vi "Get Active List - By Channel Number.vi"(7 "Parameters Array (in)":T1[](array[typedef])) -> (8 "Active Channel Numbers":i32[](array[numeric]))   [LabVIEW 2017] (continued)
"Default Value"="0"}, {"Core Number"=0, "Channel Number"=19, "Channel Name"="ENG_LB2", "Channel Speed"=100, "Label Decimal"=121, "Label Name"="Label_171", "Min Rate (mS)"=800, "Max Rate (mS)"=1200, "SDI"=0, "SSM"=3, "Create SDI"=FALSE, "Create SSM"=FALSE, "Create Parity"=FALSE, "Parameter Name"="eng_lb2_lbl171_b14_27", "Start Bit"=14, "Number of Bits"=14, "Scale"="0.015625", "Offset"="0", "Signed"=FALSE, "Unit"="% Shaftspeed", "Encoding"=enum."BNR", "Default Value"="0"}, {"Core Number"=0, "Channel Number"=19, "Channel Name"="ENG_LB2", "Channel Speed"=100, "Label Decimal"=122, "Label Name"="Label_172", "Min Rate (mS)"=800, "Max Rate (mS)"=1200, "SDI"=0, "SSM"=3, "Create SDI"=FALSE, "Create SSM"=FALSE, "Create Parity"=FALSE, "Parameter Name"="eng_lb2_lbl172_b14_27", "Start Bit"=14, "Number of Bits"=14, "Scale"="0.015625", "Offset"="0", "Signed"=FALSE, "Unit"="% Shaftspeed", "Encoding"=enum."BNR", "Default Value"="0"}, {"Core Number"=0, "Channel Number"=19, "Channel Name"="ENG_LB2", "Channel Speed"=100, "Label Decimal"=123, "Label Name"="Label_173", "Min Rate (mS)"=800, "Max Rate (mS)"=1200, "SDI"=0, "SSM"=3, "Create SDI"=FALSE, "Create SSM"=FALSE, "Create Parity"=FALSE, "Parameter Name"="eng_lb2_lbl173_b14_27", "Start Bit"=14, "Number of Bits"=14, "Scale"="0.015625", "Offset"="0", "Signed"=FALSE, "Unit"="% Shaftspeed", "Encoding"=enum."BNR", "Default Value"="0"}, {"Core Number"=0, "Channel Number"=19, "Channel Name"="ENG_LB2", "Channel Speed"=100, "Label Decimal"=124, "Label Name"="Label_174", "Min Rate (mS)"=800, "Max Rate (mS)"=1200, "SDI"=0, "SSM"=3, "Create SDI"=FALSE, "Create SSM"=FALSE, "Create Parity"=FALSE, "Parameter Name"="eng_lb2_lbl174_b14_27", "Start Bit"=14, "Number of Bits"=14, "Scale"="0.015625", "Offset"="0", "Signed"=FALSE, "Unit"="% Shaftspeed", "Encoding"=enum."BNR", "Default Value"="0"}, {"Core Number"=0, "Channel Number"=19, "Channel Name"="ENG_LB2", "Channel Speed"=100, "Label Decimal"=128, "Label Name"="Label_200", "Min Rate (mS)"=800, "Max Rate (mS)"=1200, "SDI"=0, "SSM"=3, "Create SDI"=FALSE, "Create SSM"=FALSE, "Create Parity"=FALSE, "Parameter Name"="eng_lb2_lbl200_b16_28", "Start Bit"=16, "Number of Bits"=13, "Scale"="0.125", "Offset"="0", "Signed"=TRUE, "Unit"="Degrees C", "Encoding"=enum."BNR", "Default Value"="0"}, {"Core Number"=0, "Channel Number"=19, "Channel Name"="ENG_LB2", "Channel Speed"=100, "Label Decimal"=160, "Label Name"="Label_240", "Min Rate (mS)"=800, "Max Rate (mS)"=1200, "SDI"=0, "SSM"=3, "Create SDI"=FALSE, "Create SSM"=FALSE, "Create Parity"=FALSE, "Parameter Name"="eng_lb2_lbl240_b15_28", "Start Bit"=15, "Number of Bits"=14, "Scale"="0.5", "Offset"="0", "Signed"=TRUE, "Unit"="Degrees C", "Encoding"=enum."BNR", "Default Value"="0"}, {"Core Number"=0, "Channel Number"=19, "Channel Name"="ENG_LB2", "Channel Speed"=100, "Label Decimal"=163, "Label Name"="Label_243", "Min Rate (mS)"=800, "Max Rate (mS)"=1200, "SDI"=0, "SSM"=3, "Create SDI"=FALSE, "Create SSM"=FALSE, "Create Parity"=FALSE, "Parameter Name"="eng_lb2_lbl243_b15_28", "Start Bit"=15, "Number of Bits"=14, "Scale"="0.5", "Offset"="0", "Signed"=TRUE, "Unit"="Degrees C", "Encoding"=enum."BNR", "Default Value"="0"}, {"Core Number"=0, "Channel Number"=19, "Channel Name"="ENG_LB2", "Channel Speed"=100, "Label Decimal"=72, "Label Name"="Label_110", "Min Rate (mS)"=800, "Max Rate (mS)"=1200, "SDI"=0, "SSM"=3, "Create SDI"=FALSE, "Create SSM"=FALSE, "Create Parity"=FALSE, "Parameter Name"="eng_lb2_lbl110_b20_28", "Start Bit"=20, "Number of Bits"=9, "Scale"="2", "Offset"="0", "Signed"=TRUE, "Unit"="Psig", "Encoding"=enum."BNR", "Default Value"="0"}, {"Core Number"=0, "Channel Number"=19, "Channel Name"="ENG_LB2", "Channel Speed"=100, "Label Decimal"=89, "Label Name"="Label_131", "Min Rate (mS)"=800, "Max Rate (mS)"=1200, "SDI"=0, "SSM"=3, "Create SDI"=FALSE, "Create SSM"=FALSE, "Create Parity"=FALSE, "Parameter Name"="eng_lb2_lbl131_b15_27", "Start Bit"=15, "Number of Bits"=13, "Scale"="0.015625", "Offset"="0", "Signed"=FALSE, "Unit"="Psid", "Encoding"=enum."BNR", "Default Value"="0"}, {"Core Number"=0, "Channel Number"=19, "Channel Name"="ENG_LB2", "Channel Speed"=100, "Label Decimal"=137, "Label Name"="Label_211", "Min Rate (mS)"=800, "Max Rate (mS)"=1200, "SDI"=0, "SSM"=3, "Create SDI"=FALSE, "Create SSM"=FALSE, "Create Parity"=FALSE, "Parameter Name"="eng_lb2_lbl211_b20_28", "Start Bit"=20, "Number of Bits"=9, "Scale"="0.25", "Offset"="0", "Signed"=TRUE, "Unit"="Psid", "Encoding"=enum."BNR", "Default Value"="0"}, {"Core Number"=0, "Channel Number"=19, "Channel Name"="ENG_LB2", "Channel Speed"=100, "Label Decimal"=92, "Label Name"="Label_134", "Min Rate (mS)"=800, "Max Rate (mS)"=1200, "SDI"=0, "SSM"=3, "Create SDI"=FALSE, "Create SSM"=FALSE, "Create Parity"=FALSE, "Parameter Name"="eng_lb2_lbl134_b13_28", "Start Bit"=13, "Number of Bits"=16, "Scale"="0.03125", "Offset"="0", "Signed"=TRUE, "Unit"="Degrees", "Encoding"=enum."BNR", "Default Value"="0"}, {"Core Number"=0, "Channel Number"=19, "Channel Name"="ENG_LB2", "Channel Speed"=100, "Label Decimal"=60, "Label Name"="Label_74", "Min Rate (mS)"=800, "Max Rate (mS)"=1200, "SDI"=0, "SSM"=3, "Create SDI"=FALSE, "Create SSM"=FALSE, "Create Parity"=FALSE, "Parameter Name"="eng_lb2_lbl74_b15_28", "Start Bit"=15, "Number of Bits"=14, "Scale"="0.00390625", "Offset"="0", "Signed"=TRUE, "Unit"="US pints below full", "Encoding"=enum."BNR", "Default Value"="0"}, {"Core Number"=0, "Channel Number"=19, "Channel Name"="ENG_LB2", "Channel Speed"=100, "Label Decimal"=196, "Label Name"="Label_304", "Min Rate (mS)"=800, "Max Rate (mS)"=1200, "SDI"=0, "SSM"=3, "Create SDI"=FALSE, "Create SSM"=FALSE, "Create Parity"=FALSE, "Parameter Name"="eng_lb2_lbl304_b14_28", "Start Bit"=14, "Number of Bits"=15, "Scale"="0.0078125", "Offset"="0", "Signed"=TRUE, "Unit"="Psid", "Encoding"=enum."BNR", "Default Value"="0"}, {"Core Number"=0, "Channel Number"=19, "Channel Name"="ENG_LB2", "Channel Speed"=100, "Label Decimal"=170, "Label Name"="Label_252", "Min Rate (mS)"=800, "Max Rate (mS)"=1200, "SDI"=0, "SSM"=3, "Create SDI"=FALSE, "Create SSM"=FALSE, "Create Parity"=FALSE, "Parameter Name"="eng_lb2_lbl252_b16_27", "Start Bit"=16, "Number of Bits"=12, "Scale"="0.0009765625", "Offset"="0", "Signed"=FALSE, "Unit"="Pressure ratio", "Encoding"=enum."BNR", "Default Value"="0"}, {"Core Number"=0, "Channel Number"=19, "Channel Name"="ENG_LB2", "Channel Speed"=100, "Label Decimal"=48, "Label Name"="Label_60", "Min Rate (mS)"=800, "Max Rate (mS)"=1200, "SDI"=0, "SSM"=3, "Create SDI"=FALSE, "Create SSM"=FALSE, "Create Parity"=FALSE, "Parameter Name"="eng_lb2_lbl60_b13_27", "Start Bit"=13, "Number of Bits"=15, "Scale"="1", "Offset"="0", "Signed"=FALSE, "Unit"="N/A", "Encoding"=enum."BNR", "Default Value"="0"}, {"Core Number"=0, "Channel Number"=19, "Channel Name"="ENG_LB2", "Channel Speed"=100, "Label Decimal"=150, "Label Name"="Label_226", "Min Rate (mS)"=800, "Max Rate (mS)"=1200, "SDI"=0, "SSM"=3, "Create SDI"=FALSE, "Create SSM"=FALSE, "Create Parity"=FALSE, "Parameter Name"="eng_lb2_lbl226_b13_27", "Start Bit"=13, "Number of Bits"=15, "Scale"="1", "Offset"="0", "Signed"=FALSE, "Unit"="N/A", "Encoding"=enum."BNR", "Default Value"="0"}, {"Core Number"=0, "Channel Number"=19, "Channel Name"="ENG_LB2", "Channel Speed"=100, "Label Decimal"=151, "Label Name"="Label_227", "Min Rate (mS)"=800, "Max Rate (mS)"=1200, "SDI"=0, "SSM"=3, "Create SDI"=FALSE, "Create SSM"=FALSE, "Create Parity"=FALSE, "Parameter Name"="eng_lb2_lbl227_b13_27", "Start Bit"=13, "Number of Bits"=15, "Scale"="1", "Offset"="0", "Signed"=FALSE, "Unit"="N/A", "Encoding"=enum."BNR", "Default Value"="0"}, {"Core Number"=0, "Channel Number"=19, "Channel Name"="ENG_LB2", "Channel Speed"=100, "Label Decimal"=158, "Label Name"="Label_236", "Min Rate (mS)"=800, "Max Rate (mS)"=1200, "SDI"=0, "SSM"=3, "Create SDI"=FALSE, "Create SSM"=FALSE, "Create Parity"=FALSE, "Parameter Name"="eng_lb2_lbl236_b13_27", "Start Bit"=13, "Number of Bits"=15, "Scale"="1", "Offset"="0", "Signed"=FALSE, "Unit"="N/A", "Encoding"=enum."BNR", "Default Value"="0"}, {"Core Number"=0, "Channel Number"=19, "Channel Name"="ENG_LB2", "Channel Speed"=100, "Label Decimal"=184, "Label Name"="Label_270", "Min Rate (mS)"=40, "Max Rate (mS)"=60, "SDI"=0, "SSM"=0, "Create SDI"=FALSE, "Create SSM"=FALSE, "Create Parity"=FALSE, "Parameter Name"="eng_lb2_lbl270_b10_28", "Start Bit"=10, "Number of Bits"=19, "Scale"="1", "Offset"="0", "Signed"=FALSE, "Unit"="N/A", "Encoding"=enum."Discrete", "Default Value"="0"}, {"Core Number"=0, "Channel Number"=19, "Channel Name"="ENG_LB2", "Channel Speed"=100, "Label Decimal"=232, "Label Name"="Label_350", "Min Rate (mS)"=160, "Max Rate (mS)"=240, "SDI"=0, "SSM"=0, "Create SDI"=FALSE, "Create SSM"=FALSE, "Create Parity"=FALSE, "Parameter Name"="eng_lb2_lbl350_b10_28", "Start Bit"=10, "Number of Bits"=19, "Scale"="1", "Offset"="0", "Signed"=FALSE, "Unit"="N/A", "Encoding"=enum."Discrete", "Default Value"="0"}, {"Core Number"=0, "Channel Number"=19, "Channel Name"="ENG_LB2", "Channel Speed"=100, "Label Decimal"=185, "Label Name"="Label_271", "Min Rate (mS)"=160, "Max Rate (mS)"=240, "SDI"=0, "SSM"=0, "Create SDI"=FALSE, "Create SSM"=FALSE, "Create Parity"=FALSE, "Parameter Name"="eng_lb2_lbl271_b10_28", "Start Bit"=10, "Number of Bits"=19, "Scale"="1", "Offset"="0", "Signed"=FALSE, "Unit"="N/A", "Encoding"=enum."Discrete", "Default Value"="0"}, {"Core Number"=0, "Channel Number"=19, "Channel Name"="ENG_LB2", "Channel Speed"=100, "Label Decimal"=186, "Label Name"="Label_272", "Min Rate (mS)"=160, "Max Rate (mS)"=240, "SDI"=0, "SSM"=0, "Create SDI"=FALSE, "Create SSM"=FALSE, "Create Parity"=FALSE, "Parameter Name"="eng_lb2_lbl272_b10_28", "Start Bit"=10, "Number of Bits"=19, "Scale"="1", "Offset"="0", "Signed"=FALSE, "Unit"="N/A", "Encoding"=enum."Discrete", "Default Value"="0"}, {"Core Number"=0, "Channel Number"=19, "Channel Name"="ENG_LB2", "Channel Speed"=100, "Label Decimal"=187, "Label Name"="Label_273", "Min Rate (mS)"=160, "Max Rate (mS)"=240, "SDI"=0, "SSM"=0, "Create SDI"=FALSE, "Create SSM"=FALSE, "Create Parity"=FALSE, "Parameter Name"="eng_lb2_lbl273_b10_28", "Start Bit"=10, "Number of Bits"=19, "Scale"="1", "Offset"="0", "Signed"=FALSE, "Unit"="N/A", "Encoding"=enum."Discrete", "Default Value"="0"}, {"Core Number"=0, "Channel Number"=19, "Channel Name"="ENG_LB2", "Channel Speed"=100, "Label Decimal"=188, "Label Name"="Label_274", "Min Rate (mS)"=160, "Max Rate (mS)"=240, "SDI"=0, "SSM"=0, "Create SDI"=FALSE, "Create SSM"=FALSE, "Create Parity"=FALSE, "Parameter Name"="eng_lb2_lbl274_b10_28", "Start Bit"=10, "Number of Bits"=19, "Scale"="1", "Offset"="0", "Signed"=FALSE, "Unit"="N/A", "Encoding"=enum."Discrete", "Default Value"="0"}, {"Core Number"=0, "Channel Number"=19, "Channel Name"="ENG_LB2", "Channel Speed"=100, "Label Decimal"=189, "Label Name"="Label_275", "Min Rate (mS)"=160, "Max Rate (mS)"=240, "SDI"=0, "SSM"=0, "Create SDI"=FALSE, "Create SSM"=FALSE, "Create Parity"=FALSE, "Parameter Name"="eng_lb2_lbl275_b10_28", "Start Bit"=10, "Number of Bits"=19, "Scale"="1", "Offset"="0", "Signed"=FALSE, "Unit"="N/A", "Encoding"=enum."Discrete", "Default Value"="0"}, {"Core Number"=0, "Channel Number"=19, "Channel Name"="ENG_LB2", "Channel Speed"=100, "Label Decimal"=190, "Label Name"="Label_276", "Min Rate (mS)"=160, "Max Rate (mS)"=240, "SDI"=0, "SSM"=0, "Create SDI"=FALSE, "Create SSM"=FALSE, "Create Parity"=FALSE, "Parameter Name"="eng_lb2_lbl276_b10_28", "Start Bit"=10, "Number of Bits"=19, "Scale"="1", "Offset"="0", "Signed"=FALSE, "Unit"="N/A", "Encoding"=enum."Discrete", "Default Value"="0"}, {"Core Number"=0, "Channel Number"=19, "Channel Name"="ENG_LB2", "Channel Speed"=100, "Label Decimal"=191, "Label Name"="Label_277", "Min Rate (mS)"=160, "Max Rate (mS)"=240, "SDI"=0, "SSM"=0, "Create SDI"=FALSE, "Create SSM"=FALSE, "Create Parity"=FALSE, "Parameter Name"="eng_lb2_lbl277_b10_28", "Start Bit"=10, "Number of Bits"=19, "Scale"="1", "Offset"="0", "Signed"=FALSE, "Unit"="N/A", "Encoding"=enum."Discrete", "Default Value"="0"}, {"Core Number"=0, "Channel Number"=19, "Channel Name"="ENG_LB2", "Channel Speed"=100, "Label Decimal"=254, "Label Name"="Label_376", "Min Rate (mS)"=160, "Max Rate (mS)"=240, "SDI"=0, "SSM"=0, "Create SDI"=FALSE, "Create SSM"=FALSE, "Create Parity"=FALSE, "Parameter Name"="eng_lb2_lbl376_b10_28", "Start Bit"=10, "Number of Bits"=19, "Scale"="1", "Offset"="0", "Signed"=FALSE, "Unit"="N/A", "Encoding"=enum."Discrete", "Default Value"="0"}, {"Core Number"=0, "Channel Number"=19, "Channel Name"="ENG_LB2", "Channel Speed"=100, "Label Decimal"=104, "Label Name"="Label_150", "Min Rate (mS)"=720, "Max Rate (mS)"=1080, "SDI"=0, "SSM"=0, "Create SDI"=FALSE, "Create SSM"=FALSE, "Create Parity"=FALSE, "Parameter Name"="eng_lb2_lbl150_b10_28", "Start Bit"=10, "Number of Bits"=19, "Scale"="1", "Offset"="0", "Signed"=FALSE, "Unit"="N/A", "Encoding"=enum."Discrete", "Default Value"="0"}, {"Core Number"=0, "Channel Number"=19, "Channel Name"="ENG_LB2", "Channel Speed"=100, "Label Decimal"=105, "Label Name"="Label_151", "Min Rate (mS)"=720, "Max Rate (mS)"=1080, "SDI"=0, "SSM"=0, "Create SDI"=FALSE, "Create SSM"=FALSE, "Create Parity"=FALSE, "Parameter Name"="eng_lb2_lbl151_b10_28", "Start Bit"=10, "Number of Bits"=19, "Scale"="1", "Offset"="0", "Signed"=FALSE, "Unit"="N/A", "Encoding"=enum."Discrete", "Default Value"="0"}, {"Core Number"=0, "Channel Number"=19, "Channel Name"="ENG_LB2", "Channel Speed"=100, "Label Decimal"=107, "Label Name"="Label_153", "Min Rate (mS)"=720, "Max Rate (mS)"=1080, "SDI"=0, "SSM"=0, "Create SDI"=FALSE, "Create SSM"=FALSE, "Create Parity"=FALSE, "Parameter Name"="eng_lb2_lbl153_b10_28", "Start Bit"=10, "Number of Bits"=19, "Scale"="1", "Offset"="0", "Signed"=FALSE, "Unit"="N/A", "Encoding"=enum."Discrete", "Default Value"="0"}, {"Core Number"=0, "Channel Number"=19, "Channel Name"="ENG_LB2", "Channel Speed"=100, "Label Decimal"=108, "Label Name"="Label_154", "Min Rate (mS)"=720, "Max Rate (mS)"=1080, "SDI"=0, "SSM"=0, "Create SDI"=FALSE, "Create SSM"=FALSE, "Create Parity"=FALSE, "Parameter Name"="eng_lb2_lbl154_b10_28", "Start Bit"=10, "Number of Bits"=19, "Scale"="1", "Offset"="0", "Signed"=FALSE, "Unit"="N/A", "Encoding"=enum."Discrete", "Default Value"="0"}, {"Core Number"=0, "Channel Number"=19, "Channel Name"="ENG_LB2", "Channel Speed"=100, "Label Decimal"=109, "Label Name"="Label_155", "Min Rate (mS)"=720, "Max Rate (mS)"=1080, "SDI"=0, "SSM"=0, "Create SDI"=FALSE, "Create SSM"=FALSE, "Create Parity"=FALSE, "Parameter Name"="eng_lb2_lbl155_b10_28", "Start Bit"=10, "Number of Bits"=19, "Scale"="1", "Offset"="0", "Signed"=FALSE, "Unit"="N/A", "Encoding"=enum."Discrete", "Default Value"="0"}, {"Core Number"=0, "Channel Number"=19, "Channel Name"="ENG_LB2", "Channel Speed"=100, "Label Decimal"=110, "Label Name"="Label_156", "Min Rate (mS)"=720, "Max Rate (mS)"=1080, "SDI"=0, "SSM"=0, "Create SDI"=FALSE, "Create SSM"=FALSE, "Create Parity"=FALSE, "Parameter Name"="eng_lb2_lbl156_b10_28", "Start Bit"=10, "Number of Bits"=19, "Scale"="1", "Offset"="0", "Signed"=FALSE, "Unit"="N/A", "Encoding"=enum."Discrete", "Default Value"="0"}, {"Core Number"=0, "Channel Number"=19, "Channel Name"="ENG_LB2", "Channel Speed"=100, "Label Decimal"=111, "Label Name"="Label_157", "Min Rate (mS)"=720, "Max Rate (mS)"=1080, "SDI"=0, "SSM"=0, "Create SDI"=FALSE, "Create SSM"=FALSE, "Create Parity"=FALSE, "Parameter Name"="eng_lb2_lbl157_b10_28", "Start Bit"=10, "Number of Bits"=19, "Scale"="1", "Offset"="0", "Signed"=FALSE, "Unit"="N/A", "Encoding"=enum."Discrete", "Default Value"="0"}, {"Core Number"=0, "Channel Number"=19, "Channel Name"="ENG_LB2", "Channel Speed"=100, "Label Decimal"=112, "Label Name"="Label_160", "Min Rate (mS)"=720, "Max Rate (mS)"=1080, "SDI"=0, "SSM"=0, "Create SDI"=FALSE, "Create SSM"=FALSE, "Create Parity"=FALSE, "Parameter Name"="eng_lb2_lbl160_b10_28", "Start Bit"=10, "Number of Bits"=19, "Scale"="1", "Offset"="0", "Signed"=FALSE, "Unit"="N/A", "Encoding"=enum."Discrete", "Default Value"="0"}, {"Core Number"=0, "Channel Number"=19, "Channel Name"="ENG_LB2", "Channel Speed"=100, "Label Decimal"=113, "Label Name"="Label_161", "Min Rate (mS)"=720, "Max Rate (mS)"=1080, "SDI"=0, "SSM"=0, "Create SDI"=FALSE, "Create SSM"=FALSE, "Create Parity"=FALSE, "Parameter Name"="eng_lb2_lbl161_b10_28", "Start Bit"=10, "Number of Bits"=19, "Scale"="1", "Offset"="0", "Signed"=FALSE, "Unit"="N/A", "Encoding"=enum."Discrete", "Default Value"="0"}, {"Core Number"=0, "Channel Number"=19, "Channel Name"="ENG_LB2", "Channel Speed"=100, "Label Decimal"=114, "Label Name"="Label_162", "Min Rate (mS)"=720, "Max Rate (mS)"=1080, "SDI"=0, "SSM"=0, "Create SDI"=FALSE, "Create SSM"=FALSE, "Create Parity"=FALSE, "Parameter Name"="eng_lb2_lbl162_b10_28", "Start Bit"=10, "Number of Bits"=19, "Scale"="1", "Offset"="0", "Signed"=FALSE, "Unit"="N/A", "Encoding"=enum."Discrete", "Default Value"="0"}, {"Core Number"=0, "Channel Number"=19, "Channel Name"="ENG_LB2", "Channel Speed"=100, "Label Decimal"=115, "Label Name"="Label_163", "Min Rate (mS)"=720, "Max Rate (mS)"=1080, "SDI"=0, "SSM"=0, "Create SDI"=FALSE, "Create SSM"=FALSE, "Create Parity"=FALSE, "Parameter Name"="eng_lb2_lbl163_b10_28", "Start Bit"=10, "Number of Bits"=19, "Scale"="1", "Offset"="0", "Signed"=FALSE, "Unit"="N/A", "Encoding"=enum."Discrete", "Default Value"="0"}, {"Core Number"=0, "Channel Number"=19, "Channel Name"="ENG_LB2", "Channel Speed"=100, "Label Decimal"=117, "Label Name"="Label_165", "Min Rate (mS)"=720, "Max Rate (mS)"=1080, "SDI"=0, "SSM"=0, "Create SDI"=FALSE, "Create SSM"=FALSE, "Create Parity"=FALSE, "Parameter Name"="eng_lb2_lbl165_b10_28", "Start Bit"=10, "Number of Bits"=19, "Scale"="1", "Offset"="0", "Signed"=FALSE, "Unit"="N/A", "Encoding"=enum."Discrete", "Default Value"="0"}, {"Core Number"=0, "Channel Number"=19, "Channel Name"="ENG_LB2", "Channel Speed"=100, "Label Decimal"=119, "Label Name"="Label_167", "Min Rate (mS)"=720, "Max Rate (mS)"=1080, "SDI"=0, "SSM"=0, "Create SDI"=FALSE, "Create SSM"=FALSE, "Create Parity"=FALSE, "Parameter Name"="eng_lb2_lbl167_b10_28", "Start Bit"=10, "Number of Bits"=19, "Scale"="1", "Offset"="0", "Signed"=FALSE, "Unit"="N/A", "Encoding"=enum."Discrete", "Default Value"="0"}, {"Core Number"=0, "Channel Number"=19, "Channel Name"="ENG_LB2", "Channel Speed"=100, "Label Decimal"=120, "Label Name"="Label_170", "Min Rate (mS)"=720, "Max Rate (mS)"=1080, "SDI"=0, "SSM"=0, "Create SDI"=FALSE, "Create SSM"=FALSE, "Create Parity"=FALSE, "Parameter Name"="eng_lb2_lbl170_b10_28", "Start Bit"=10, "Number of Bits"=19, "Scale"="1", "Offset"="0", "Signed"=FALSE, "Unit"="N/A", "Encoding"=enum."Discrete", "Default Value"="0"}, {"Core Number"=0, "Channel Number"=19, "Channel Name"="ENG_LB2", "Channel Speed"=100, "Label Decimal"=125, "Label Name"="Label_175", "Min Rate (mS)"=720, "Max Rate (mS)"=1080, "SDI"=0, "SSM"=0, "Create SDI"=FALSE, "Create SSM"=FALSE, "Create Parity"=FALSE, "Parameter Name"="eng_lb2_lbl175_b10_28", "Start Bit"=10, "Number of Bits"=19, "Scale"="1", "Offset"="0", "Signed"=FALSE, "Unit"="N/A", "Encoding"=enum."Discrete", "Default Value"="0"}, {"Core Number"=0, "Channel Number"=19, "Channel Name"="ENG_LB2", "Channel Speed"=100, "Label Decimal"=126, "Label Name"="Label_176", "Min Rate (mS)"=720, "Max Rate (mS)"=1080, "SDI"=0, "SSM"=0, "Create SDI"=FALSE, "Create SSM"=FALSE, "Create Parity"=FALSE, "Parameter Name"="eng_lb2_lbl176_b10_28", "Start Bit"=10, "Number of Bits"=19, "Scale"="1", "Offset"="0", "Signed"=FALSE, "Unit"="N/A", "Encoding"=enum."Discrete", "Default Value"="0"}, {"Core Number"=0, "Channel Number"=19, "Channel Name"="ENG_LB2", "Channel Speed"=100, "Label Decimal"=127, "Label Name"="Label_177", "Min Rate (mS)"=720, "Max Rate (mS)"=1080, "SDI"=0, "SSM"=0, "Create SDI"=FALSE, "Create SSM"=FALSE, "Create Parity"=FALSE, "Parameter Name"="eng_lb2_lbl177_b10_28", "Start Bit"=10, "Number of Bits"=19, "Scale"="1", "Offset"="0", "Signed"=FALSE, "Unit"="N/A", "Encoding"=enum."Discrete", "Default Value"="0"}, {"Core Number"=0, "Channel Number"=19, "Channel Name"="ENG_LB2", "Channel Speed"=100, "Label Decimal"=129, "Label Name"="Label_201", "Min Rate (mS)"=720, "Max Rate (mS)"=1080, "SDI"=0, "SSM"=0, "Create SDI"=FALSE, "Create SSM"=FALSE, "Create Parity"=FALSE, "Parameter Name"="eng_lb2_lbl201_b10_28", "Start Bit"=10, "Number of Bits"=19, "Scale"="1", "Offset"="0", "Signed"=FALSE, "Unit"="N/A", "Encoding"=enum."Discrete", "Default Value"="0"}, {"Core Number"=0, "Channel Number"=19, "Channel Name"="ENG_LB2", "Channel Speed"=100, "Label Decimal"=130, "Label Name"="Label_202", "Min Rate (mS)"=720, "Max Rate (mS)"=1080, "SDI"=0, "SSM"=0, "Create SDI"=FALSE, "Create SSM"=FALSE, "Create Parity"=FALSE, "Parameter Name"="eng_lb2_lbl202_b10_28", "Start Bit"=10, "Number of Bits"=19, "Scale"="1", "Offset"="0", "Signed"=FALSE, "Unit"="N/A", "Encoding"=enum."Discrete", "Default Value"="0"}, {"Core Number"=0, "Channel Number"=19, "Channel Name"="ENG_LB2", "Channel Speed"=100, "Label Decimal"=132, "Label Name"="Label_204", "Min Rate (mS)"=720, "Max Rate (mS)"=1080, "SDI"=0, "SSM"=0, "Create SDI"=FALSE, "Create SSM"=FALSE, "Create Parity"=FALSE, "Parameter Name"="eng_lb2_lbl204_b10_28", "Start Bit"=10, "Number of Bits"=19, "Scale"="1", "Offset"="0", "Signed"=FALSE, "Unit"="N/A", "Encoding"=enum."Discrete", "Default Value"="0"}, {"Core Number"=0, "Channel Number"=19, "Channel Name"="ENG_LB2", "Channel Speed"=100, "Label Decimal"=139, "Label Name"="Label_213", "Min Rate (mS)"=800, "Max Rate (mS)"=1200, "SDI"=0, "SSM"=0, "Create SDI"=FALSE, "Create SSM"=FALSE, "Create Parity"=FALSE, "Parameter Name"="eng_lb2_lbl213_b10_28", "Start Bit"=10, "Number of Bits"=19, "Scale"="1", "Offset"="0", "Signed"=FALSE, "Unit"="N/A", "Encoding"=enum."Discrete", "Default Value"="0"}, {"Core Number"=0, "Channel Number"=19, "Channel Name"="ENG_LB2", "Channel Speed"=100, "Label Decimal"=64, "Label Name"="Label_100", "Min Rate (mS)"=800, "Max Rate (mS)"=1200, "SDI"=0, "SSM"=0, "Create SDI"=FALSE, "Create SSM"=FALSE, "Create Parity"=FALSE, "Parameter Name"="eng_lb2_lbl100_b13_27", "Start Bit"=13, "Number of Bits"=15, "Scale"="1", "Offset"="0", "Signed"=FALSE, "Unit"="N/A", "Encoding"=enum."Discrete", "Default Value"="0"}, {"Core Number"=0, "Channel Number"=19, "Channel Name"="ENG_LB2", "Channel Speed"=100, "Label Decimal"=66, "Label Name"="Label_102", "Min Rate (mS)"=800, "Max Rate (mS)"=1200, "SDI"=0, "SSM"=0, "Create SDI"=FALSE, "Create SSM"=FALSE, "Create Parity"=FALSE, "Parameter Name"="eng_lb2_lbl102_b13_27", "Start Bit"=13, "Number of Bits"=15, "Scale"="1", "Offset"="0", "Signed"=FALSE, "Unit"="N/A", "Encoding"=enum."Discrete", "Default Value"="0"}, {"Core Number"=0, "Channel Number"=20, "Channel Name"="ENG_RA1", "Channel Speed"=100, "Label Decimal"=224, "Label Name"="Label_340", "Min Rate (mS)"=40, "Max Rate (mS)"=60, "SDI"=3, "SSM"=3, "Create SDI"=FALSE, "Create SSM"=FALSE, "Create Parity"=FALSE, "Parameter Name"="eng_ra1_lbl340_b15_27", "Start Bit"=15, "Number of Bits"=13, "Scale"="0.00048828125", "Offset"="0", "Signed"=FALSE, "Unit"="Pressure ratio", "Encoding"=enum."BNR", "Default Value"="0"}, {"Core Number"=0, "Channel Number"=20, "Channel Name"="ENG_RA1", "Channel Speed"=100, "Label Decimal"=226, "Label Name"="Label_342", "Min Rate (mS)"=40, "Max Rate (mS)"=60, "SDI"=3, "SSM"=3, "Create SDI"=FALSE, "Create SSM"=FALSE, "Create Parity"=FALSE, "Parameter Name"="eng_ra1_lbl342_b15_27", "Start Bit"=15, "Number of Bits"=13, "Scale"="0.00048828125", "Offset"="0", "Signed"=FALSE, "Unit"="Pressure ratio", "Encoding"=enum."BNR", "Default Value"="0"}, {"Core Number"=0, "Channel Number"=20, "Channel Name"="ENG_RA1", "Channel Speed"=100, "Label Decimal"=180, "Label Name"="Label_264", "Min Rate (mS)"=40, "Max Rate (mS)"=60, "SDI"=3, "SSM"=3, "Create SDI"=FALSE, "Create SSM"=FALSE, "Create Parity"=FALSE, "Parameter Name"="eng_ra1_lbl264_b14_27", "Start Bit"=14, "Number of Bits"=14, "Scale"="0.0625", "Offset"="0", "Signed"=FALSE, "Unit"="Psia", "Encoding"=enum."BNR", "Default Value"="0"}, {"Core Number"=0, "Channel Number"=20, "Channel Name"="ENG_RA1", "Channel Speed"=100, "Label Decimal"=193, "Label Name"="Label_301", "Min Rate (mS)"=40, "Max Rate (mS)"=60, "SDI"=3, "SSM"=3, "Create SDI"=FALSE, "Create SSM"=FALSE, "Create Parity"=FALSE, "Parameter Name"="eng_ra1_lbl301_b17_28", "Start Bit"=17, "Number of Bits"=12, "Scale"="0.0625", "Offset"="0", "Signed"=TRUE, "Unit"="Percentage", "Encoding"=enum."BNR", "Default Value"="0"}, {"Core Number"=0, "Channel Number"=20, "Channel Name"="ENG_RA1", "Channel Speed"=100, "Label Decimal"=212, "Label Name"="Label_324", "Min Rate (mS)"=40, "Max Rate (mS)"=60, "SDI"=3, "SSM"=3, "Create SDI"=FALSE, "Create SSM"=FALSE, "Create Parity"=FALSE, "Parameter Name"="eng_ra1_lbl324_b14_28", "Start Bit"=14, "Number of Bits"=15, "Scale"="0.125", "Offset"="0", "Signed"=TRUE, "Unit"="Percentage", "Encoding"=enum."BNR", "Default Value"="0"}, {"Core Number"=0, "Channel Number"=20, "Channel Name"="ENG_RA1", "Channel Speed"=100, "Label Decimal"=91, "Label Name"="Label_133", "Min Rate (mS)"=40, "Max Rate (mS)"=60, "SDI"=3, "SSM"=3, "Create SDI"=FALSE, "Create SSM"=FALSE, "Create Parity"=FALSE, "Parameter Name"="eng_ra1_lbl133_b16_28", "Start Bit"=16, "Number of Bits"=13, "Scale"="0.0439453125", "Offset"="0", "Signed"=TRUE, "Unit"="Degrees", "Encoding"=enum."BNR", "Default Value"="0"}, {"Core Number"=0, "Channel Number"=20, "Channel Name"="ENG_RA1", "Channel Speed"=100, "Label Decimal"=228, "Label Name"="Label_344", "Min Rate (mS)"=40, "Max Rate (mS)"=60, "SDI"=3, "SSM"=3, "Create SDI"=FALSE, "Create SSM"=FALSE, "Create Parity"=FALSE, "Parameter Name"="eng_ra1_lbl344_b13_27", "Start Bit"=13, "Number of Bits"=15, "Scale"="0.0078125", "Offset"="0", "Signed"=FALSE, "Unit"="% Shaftspeed", "Encoding"=enum."BNR", "Default Value"="0"}, {"Core Number"=0, "Channel Number"=20, "Channel Name"="ENG_RA1", "Channel Speed"=100, "Label Decimal"=230, "Label Name"="Label_346", "Min Rate (mS)"=40, "Max Rate (mS)"=60, "SDI"=3, "SSM"=3, "Create SDI"=FALSE, "Create SSM"=FALSE, "Create Parity"=FALSE, "Parameter Name"="eng_ra1_lbl346_b13_27", "Start Bit"=13, "Number of Bits"=15, "Scale"="0.0078125", "Offset"="0", "Signed"=FALSE, "Unit"="% Shaftspeed", "Encoding"=enum."BNR", "Default Value"="0"}, {"Core Number"=0, "Channel Number"=20, "Channel Name"="ENG_RA1", "Channel Speed"=100, "Label Decimal"=118, "Label Name"="Label_166", "Min Rate (mS)"=40, "Max Rate (mS)"=60, "SDI"=3, "SSM"=3, "Create SDI"=FALSE, "Create SSM"=FALSE, "Create Parity"=FALSE, "Parameter Name"="eng_ra1_lbl166_b16_27", "Start Bit"=16, "Number of Bits"=12, "Scale"="0.0009765625", "Offset"="0", "Signed"=FALSE, "Unit"="Pressure ratio", "Encoding"=enum."BNR", "Default Value"="0"}, {"Core Number"=0, "Channel Number"=20, "Channel Name"="ENG_RA1", "Channel Speed"=100, "Label Decimal"=172, "Label Name"="Label_254", "Min Rate (mS)"=40, "Max Rate (mS)"=60, "SDI"=3, "SSM"=3, "Create SDI"=FALSE, "Create SSM"=FALSE, "Create Parity"=FALSE, "Parameter Name"="eng_ra1_lbl254_b14_27", "Start Bit"=14, "Number of Bits"=14, "Scale"="0.015625", "Offset"="0", "Signed"=FALSE, "Unit"="% Shaftspeed", "Encoding"=enum."BNR", "Default Value"="0"}, {"Core Number"=0, "Channel Number"=20, "Channel Name"="ENG_RA1", "Channel Speed"=100, "Label Decimal"=222, "Label Name"="Label_336", "Min Rate (mS)"=40, "Max Rate (mS)"=60, "SDI"=3, "SSM"=3, "Create SDI"=FALSE, "Create SSM"=FALSE, "Create Parity"=FALSE, "Parameter Name"="eng_ra1_lbl336_b14_27", "Start Bit"=14, "Number of Bits"=14, "Scale"="0.015625", "Offset"="0", "Signed"=FALSE, "Unit"="% Shaftspeed", "Encoding"=enum."BNR", "Default Value"="0"}, {"Core Number"=0, "Channel Number"=20, "Channel Name"="ENG_RA1", "Channel Speed"=100, "Label Decimal"=225, "Label Name"="Label_341", "Min Rate (mS)"=40, "Max Rate (mS)"=60, "SDI"=3, "SSM"=3, "Create SDI"=FALSE, "Create SSM"=FALSE, "Create Parity"=FALSE, "Parameter Name"="eng_ra1_lbl341_b15_27", "Start Bit"=15, "Number of Bits"=13, "Scale"="0.00048828125", "Offset"="0", "Signed"=FALSE, "Unit"="Pressure ratio", "Encoding"=enum."BNR", "Default Value"="0"}, {"Core Number"=0, "Channel Number"=20, "Channel Name"="ENG_RA1", "Channel Speed"=100, "Label Decimal"=227, "Label Name"="Label_343", "Min Rate (mS)"=40, "Max Rate (mS)"=60, "SDI"=3, "SSM"=3, "Create SDI"=FALSE, "Create SSM"=FALSE, "Create Parity"=FALSE, "Parameter Name"="eng_ra1_lbl343_b14_27", "Start Bit"=14, "Number of Bits"=14, "Scale"="0.015625", "Offset"="0", "Signed"=FALSE, "Unit"="% Shaftspeed", "Encoding"=enum."BNR", "Default Value"="0"}, {"Core Number"=0, "Channel Number"=20, "Channel Name"="ENG_RA1", "Channel Speed"=100, "Label Decimal"=74, "Label Name"="Label_112", "Min Rate (mS)"=40, "Max Rate (mS)"=60, "SDI"=3, "SSM"=3, "Create SDI"=FALSE, "Create SSM"=FALSE, "Create Parity"=FALSE, "Parameter Name"="eng_ra1_lbl112_b17_28", "Start Bit"=17, "Number of Bits"=12, "Scale"="0.015625", "Offset"="0", "Signed"=TRUE, "Unit"="Percentage", "Encoding"=enum."BNR", "Default Value"="0"}, {"Core Number"=0, "Channel Number"=20, "Channel Name"="ENG_RA1", "Channel Speed"=100, "Label Decimal"=166, "Label Name"="Label_246", "Min Rate (mS)"=40, "Max Rate (mS)"=60, "SDI"=3, "SSM"=3, "Create SDI"=FALSE, "Create SSM"=FALSE, "Create Parity"=FALSE, "Parameter Name"="eng_ra1_lbl246_b17_28", "Start Bit"=17, "Number of Bits"=12, "Scale"="0.0625", "Offset"="0", "Signed"=TRUE, "Unit"="Percentage", "Encoding"=enum."BNR", "Default Value"="0"}, {"Core Number"=0, "Channel Number"=20, "Channel Name"="ENG_RA1", "Channel Speed"=100, "Label Decimal"=194, "Label Name"="Label_302", "Min Rate (mS)"=40, "Max Rate (mS)"=60, "SDI"=3, "SSM"=3, "Create SDI"=FALSE, "Create SSM"=FALSE, "Create Parity"=FALSE, "Parameter Name"="eng_ra1_lbl302_b17_28", "Start Bit"=17, "Number of Bits"=12, "Scale"="0.0625", "Offset"="0", "Signed"=TRUE, "Unit"="Percentage", "Encoding"=enum."BNR", "Default Value"="0"}, {"Core Number"=0, "Channel Number"=20, "Channel Name"="ENG_RA1", "Channel Speed"=100, "Label Decimal"=211, "Label Name"="Label_323", "Min Rate (mS)"=40, "Max Rate (mS)"=60, "SDI"=3, "SSM"=3, "Create SDI"=FALSE, "Create SSM"=FALSE, "Create Parity"=FALSE, "Parameter Name"="eng_ra1_lbl323_b14_28", "Start Bit"=14, "Number of Bits"=15, "Scale"="0.0625", "Offset"="0", "Signed"=TRUE, "Unit"="Percentage", "Encoding"=enum."BNR", "Default Value"="0"}, {"Core Number"=0, "Channel Number"=20, "Channel Name"="ENG_RA1", "Channel Speed"=100, "Label Decimal"=90, "Label Name"="Label_132", "Min Rate (mS)"=80, "Max Rate (mS)"=120, "SDI"=3, "SSM"=3, "Create SDI"=FALSE, "Create SSM"=FALSE, "Create Parity"=FALSE, "Parameter Name"="eng_ra1_lbl132_b14_27", "Start Bit"=14, "Number of Bits"=14, "Scale"="0.00390625", "Offset"="0", "Signed"=FALSE, "Unit"="Psia", "Encoding"=enum."BNR", "Default Value"="0"}, {"Core Number"=0, "Channel Number"=20, "Channel Name"="ENG_RA1", "Channel Speed"=100, "Label Decimal"=181, "Label Name"="Label_265", "Min Rate (mS)"=80, "Max Rate (mS)"=120, "SDI"=3, "SSM"=3, "Create SDI"=FALSE, "Create SSM"=FALSE, "Create Parity"=FALSE, "Parameter Name"="eng_ra1_lbl265_b16_28", "Start Bit"=16, "Number of Bits"=13, "Scale"="0.5", "Offset"="0", "Signed"=TRUE, "Unit"="Degrees C", "Encoding"=enum."BNR", "Default Value"="0"}, {"Core Number"=0, "Channel Number"=20, "Channel Name"="ENG_RA1", "Channel Speed"=100, "Label Decimal"=208, "Label Name"="Label_320", "Min Rate (mS)"=80, "Max Rate (mS)"=120, "SDI"=3, "SSM"=3, "Create SDI"=FALSE, "Create SSM"=FALSE, "Create Parity"=FALSE, "Parameter Name"="eng_ra1_lbl320_b16_28", "Start Bit"=16, "Number of Bits"=13, "Scale"="0.5", "Offset"="0", "Signed"=TRUE, "Unit"="Degrees C", "Encoding"=enum."BNR", "Default Value"="0"}, {"Core Number"=0, "Channel Number"=20, "Channel Name"="ENG_RA1", "Channel Speed"=100, "Label Decimal"=209, "Label Name"="Label_321", "Min Rate (mS)"=80, "Max Rate (mS)"=120, "SDI"=3, "SSM"=3, "Create SDI"=FALSE, "Create SSM"=FALSE, "Create Parity"=FALSE, "Parameter Name"="eng_ra1_lbl321_b16_28", "Start Bit"=16, "Number of Bits"=13, "Scale"="0.5", "Offset"="0", "Signed"=TRUE, "Unit"="Degrees C", "Encoding"=enum."BNR", "Default Value"="0"}, {"Core Number"=0, "Channel Number"=20, "Channel Name"="ENG_RA1", "Channel Speed"=100, "Label Decimal"=229, "Label Name"="Label_345", "Min Rate (mS)"=80, "Max Rate (mS)"=120, "SDI"=3, "SSM"=3, "Create SDI"=FALSE, "Create SSM"=FALSE, "Create Parity"=FALSE, "Parameter Name"="eng_ra1_lbl345_b15_28", "Start Bit"=15, "Number of Bits"=14, "Scale"="0.5", "Offset"="0", "Signed"=TRUE, "Unit"="Degrees C", "Encoding"=enum."BNR", "Default Value"="0"}, {"Core Number"=0, "Channel Number"=20, "Channel Name"="ENG_RA1", "Channel Speed"=100, "Label Decimal"=252, "Label Name"="Label_374", "Min Rate (mS)"=80, "Max Rate (mS)"=120, "SDI"=3, "SSM"=3, "Create SDI"=FALSE, "Create SSM"=FALSE, "Create Parity"=FALSE, "Parameter Name"="eng_ra1_lbl374_b16_28", "Start Bit"=16, "Number of Bits"=13, "Scale"="0.03125", "Offset"="0", "Signed"=TRUE, "Unit"="% Deployed", "Encoding"=enum."BNR", "Default Value"="0"}, {"Core Number"=0, "Channel Number"=20, "Channel Name"="ENG_RA1", "Channel Speed"=100, "Label Decimal"=253, "Label Name"="Label_375", "Min Rate (mS)"=80, "Max Rate (mS)"=120, "SDI"=3, "SSM"=3, "Create SDI"=FALSE, "Create SSM"=FALSE, "Create Parity"=FALSE, "Parameter Name"="eng_ra1_lbl375_b16_28", "Start Bit"=16, "Number of Bits"=13, "Scale"="0.03125", "Offset"="0", "Signed"=TRUE, "Unit"="% Deployed", "Encoding"=enum."BNR", "Default Value"="0"}, {"Core Number"=0, "Channel Number"=20, "Channel Name"="ENG_RA1", "Channel Speed"=100, "Label Decimal"=75, "Label Name"="Label_113", "Min Rate (mS)"=160, "Max Rate (mS)"=240, "SDI"=3, "SSM"=3, "Create SDI"=FALSE, "Create SSM"=FALSE, "Create Parity"=FALSE, "Parameter Name"="eng_ra1_lbl113_b14_27", "Start Bit"=14, "Number of Bits"=14, "Scale"="0.0009765625", "Offset"="0", "Signed"=FALSE, "Unit"="IPS", "Encoding"=enum."BNR", "Default Value"="0"}, {"Core Number"=0, "Channel Number"=20, "Channel Name"="ENG_RA1", "Channel Speed"=100, "Label Decimal"=78, "Label Name"="Label_116", "Min Rate (mS)"=160, "Max Rate (mS)"=240, "SDI"=3, "SSM"=3, "Create SDI"=FALSE, "Create SSM"=FALSE, "Create Parity"=FALSE, "Parameter Name"="eng_ra1_lbl116_b14_27", "Start Bit"=14, "Number of Bits"=14, "Scale"="0.0009765625", "Offset"="0", "Signed"=FALSE, "Unit"="IPS", "Encoding"=enum."BNR", "Default Value"="0"}, {"Core Number"=0, "Channel Number"=20, "Channel Name"="ENG_RA1", "Channel Speed"=100, "Label Decimal"=79, "Label Name"="Label_117", "Min Rate (mS)"=160, "Max Rate (mS)"=240, "SDI"=3, "SSM"=3, "Create SDI"=FALSE, "Create SSM"=FALSE, "Create Parity"=FALSE, "Parameter Name"="eng_ra1_lbl117_b14_27", "Start Bit"=14, "Number of Bits"=14, "Scale"="0.0009765625", "Offset"="0", "Signed"=FALSE, "Unit"="IPS", "Encoding"=enum."BNR", "Default Value"="0"}, {"Core Number"=0, "Channel Number"=20, "Channel Name"="ENG_RA1", "Channel Speed"=100, "Label Decimal"=80, "Label Name"="Label_120", "Min Rate (mS)"=160, "Max Rate (mS)"=240, "SDI"=3, "SSM"=3, "Create SDI"=FALSE, "Create SSM"=FALSE, "Create Parity"=FALSE, "Parameter Name"="eng_ra1_lbl120_b14_27", "Start Bit"=14, "Number of Bits"=14, "Scale"="0.0009765625", "Offset"="0", "Signed"=FALSE, "Unit"="IPS", "Encoding"=enum."BNR", "Default Value"="0"}, {"Core Number"=0, "Channel Number"=20, "Channel Name"="ENG_RA1", "Channel Speed"=100, "Label Decimal"=81, "Label Name"="Label_121", "Min Rate (mS)"=160, "Max Rate (mS)"=240, "SDI"=3, "SSM"=3, "Create SDI"=FALSE, "Create SSM"=FALSE, "Create Parity"=FALSE, "Parameter Name"="eng_ra1_lbl121_b14_27", "Start Bit"=14, "Number of Bits"=14, "Scale"="0.0009765625", "Offset"="0", "Signed"=FALSE, "Unit"="IPS", "Encoding"=enum."BNR", "Default Value"="0"}, {"Core Number"=0, "Channel Number"=20, "Channel Name"="ENG_RA1", "Channel Speed"=100, "Label Decimal"=82, "Label Name"="Label_122", "Min Rate (mS)"=160, "Max Rate (mS)"=240, "SDI"=3, "SSM"=3, "Create SDI"=FALSE, "Create SSM"=FALSE, "Create Parity"=FALSE, "Parameter Name"="eng_ra1_lbl122_b14_27", "Start Bit"=14, "Number of Bits"=14, "Scale"="0.0009765625", "Offset"="0", "Signed"=FALSE, "Unit"="IPS", "Encoding"=enum."BNR", "Default Value"="0"}, {"Core Number"=0, "Channel Number"=20, "Channel Name"="ENG_RA1", "Channel Speed"=100, "Label Decimal"=83, "Label Name"="Label_123", "Min Rate (mS)"=160, "Max Rate (mS)"=240, "SDI"=3, "SSM"=3, "Create SDI"=FALSE, "Create SSM"=FALSE, "Create Parity"=FALSE, "Parameter Name"="eng_ra1_lbl123_b13_27", "Start Bit"=13, "Number of Bits"=15, "Scale"="0.0078125", "Offset"="0", "Signed"=FALSE, "Unit"="% Shaftspeed", "Encoding"=enum."BNR", "Default Value"="0"}, {"Core Number"=0, "Channel Number"=20, "Channel Name"="ENG_RA1", "Channel Speed"=100, "Label Decimal"=84, "Label Name"="Label_124", "Min Rate (mS)"=160, "Max Rate (mS)"=240, "SDI"=3, "SSM"=3, "Create SDI"=FALSE, "Create SSM"=FALSE, "Create Parity"=FALSE, "Parameter Name"="eng_ra1_lbl124_b13_27", "Start Bit"=13, "Number of Bits"=15, "Scale"="0.0078125", "Offset"="0", "Signed"=FALSE, "Unit"="% Shaftspeed", "Encoding"=enum."BNR", "Default Value"="0"}, {"Core Number"=0, "Channel Number"=20, "Channel Name"="ENG_RA1", "Channel Speed"=100, "Label Decimal"=87, "Label Name"="Label_127", "Min Rate (mS)"=160, "Max Rate (mS)"=240, "SDI"=3, "SSM"=3, "Create SDI"=FALSE, "Create SSM"=FALSE, "Create Parity"=FALSE, "Parameter Name"="eng_ra1_lbl127_b19_27", "Start Bit"=19, "Number of Bits"=9, "Scale"="1", "Offset"="0", "Signed"=FALSE, "Unit"="Deg", "Encoding"=enum."BNR", "Default Value"="0"}, {"Core Number"=0, "Channel Number"=20, "Channel Name"="ENG_RA1", "Channel Speed"=100, "Label Decimal"=93, "Label Name"="Label_135", "Min Rate (mS)"=160, "Max Rate (mS)"=240, "SDI"=3, "SSM"=3, "Create SDI"=FALSE, "Create SSM"=FALSE, "Create Parity"=FALSE, "Parameter Name"="eng_ra1_lbl135_b19_27", "Start Bit"=19, "Number of Bits"=9, "Scale"="1", "Offset"="0", "Signed"=FALSE, "Unit"="Deg", "Encoding"=enum."BNR", "Default Value"="0"}, {"Core Number"=0, "Channel Number"=20, "Channel Name"="ENG_RA1", "Channel Speed"=100, "Label Decimal"=94, "Label Name"="Label_136", "Min Rate (mS)"=160, "Max Rate (mS)"=240, "SDI"=3, "SSM"=3, "Create SDI"=FALSE, "Create SSM"=FALSE, "Create Parity"=FALSE, "Parameter Name"="eng_ra1_lbl136_b19_27", "Start Bit"=19, "Number of Bits"=9, "Scale"="1", "Offset"="0", "Signed"=FALSE, "Unit"="Deg", "Encoding"=enum."BNR", "Default Value"="0"}, {"Core Number"=0, "Channel Number"=20, "Channel Name"="ENG_RA1", "Channel Speed"=100, "Label Decimal"=95, "Label Name"="Label_137", "Min Rate (mS)"=160, "Max Rate (mS)"=240, "SDI"=3, "SSM"=3, "Create SDI"=FALSE, "Create SSM"=FALSE, "Create Parity"=FALSE, "Parameter Name"="eng_ra1_lbl137_b19_27", "Start Bit"=19, "Number of Bits"=9, "Scale"="1", "Offset"="0", "Signed"=FALSE, "Unit"="Deg", "Encoding"=enum."BNR", "Default Value"="0"}, {"Core Number"=0, "Channel Number"=20, "Channel Name"="ENG_RA1", "Channel Speed"=100, "Label Decimal"=77, "Label Name"="Label_115", "Min Rate (mS)"=160, "Max Rate (mS)"=240, "SDI"=3, "SSM"=3, "Create SDI"=FALSE, "Create SSM"=FALSE, "Create Parity"=FALSE, "Parameter Name"="eng_ra1_lbl115_b17_28", "Start Bit"=17, "Number of Bits"=12, "Scale"="0.25", "Offset"="0", "Signed"=TRUE, "Unit"="Degrees C", "Encoding"=enum."BNR", "Default Value"="0"}, {"Core Number"=0, "Channel Number"=20, "Channel Name"="ENG_RA1", "Channel Speed"=100, "Label Decimal"=164, "Label Name"="Label_244", "Min Rate (mS)"=160, "Max Rate (mS)"=240, "SDI"=3, "SSM"=3, "Create SDI"=FALSE, "Create SSM"=FALSE, "Create Parity"=FALSE, "Parameter Name"="eng_ra1_lbl244_b12_27", "Start Bit"=12, "Number of Bits"=16, "Scale"="0.25", "Offset"="0", "Signed"=FALSE, "Unit"="pph", "Encoding"=enum."BNR", "Default Value"="0"}, {"Core Number"=0, "Channel Number"=20, "Channel Name"="ENG_RA1", "Channel Speed"=100, "Label Decimal"=206, "Label Name"="Label_316", "Min Rate (mS)"=160, "Max Rate (mS)"=240, "SDI"=3, "SSM"=3, "Create SDI"=FALSE, "Create SSM"=FALSE, "Create Parity"=FALSE, "Parameter Name"="eng_ra1_lbl316_b16_28", "Start Bit"=16, "Number of Bits"=13, "Scale"="0.25", "Offset"="0", 
